vi "Exercise_3-8_Liam_Hubbard.vi"() -> ()   [LabVIEW 2014]
panel:
  in  "Current Temp":dbl
  in  "Max Temp":dbl
  in  "Min Temp":dbl
  out "Warning Text":string
  out "Warning?":bool
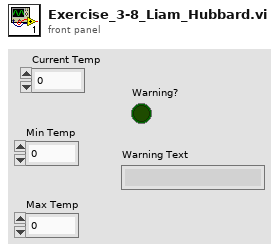
[diagram p1: front panel]
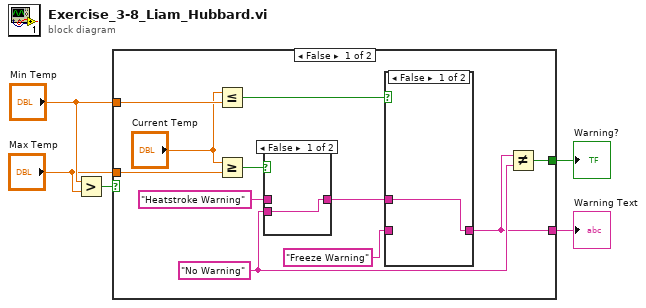
[diagram p0: block diagram]
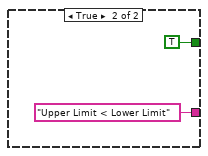
[diagram p4: hidden frame]
diagram:
  n1 = Greater?(x="Min Temp", y="Max Temp") -> (0:w5:bool)
  n2 = case shown="False" w5 {
    tunnel: "Min Temp" -> [w14 _]
    tunnel: "Max Temp" -> [w16 _]
    tunnel: [w6 "Upper Limit < Lower Limit"] -> w2
    tunnel: [w15 TRUE] -> w1
    frame False {
      w10 = "No Warning"
      n3 = Less Or Equal?(x="Current Temp", y=w14) -> (x <= y?=w7:bool)
      n4 = Greater Or Equal?(x="Current Temp", y=w16) -> (x >= y?=w12:bool)
      n5 = case shown="False" w12 {
        tunnel: "Heatstroke Warning" ("t") -> [_ w20]
        tunnel: w10 -> [w19 _]
        tunnel: [w19 w20] -> w9
        frame False {
        }
        frame True {
        }
      }
      n6 = case shown="False" w7 {
        tunnel: w9 -> [w17 _]
        tunnel: "Freeze Warning" -> [_ w18]
        tunnel: [w17 w18] -> w6
        frame False {
        }
        frame True {
        }
      }
      n7 = Not Equal?(x=w6, y=w10) -> (x != y?=w15:bool)
    }
    frame True {
    }
  }
  "Warning Text" <- w2
  "Warning?" <- w1
